vi "create.vi"(8 "error in (no error)":errorcluster) -> (0 "error out":errorcluster, 3 "system out":refnum<class "system.lvclass">)   [LabVIEW 2021, in "system.lvclass"]
uses:
  system.lvclass
  system.lvclass/system.ctl
  system.threading/system.threading.lvclass
  system.logging/system.logging.lvclass
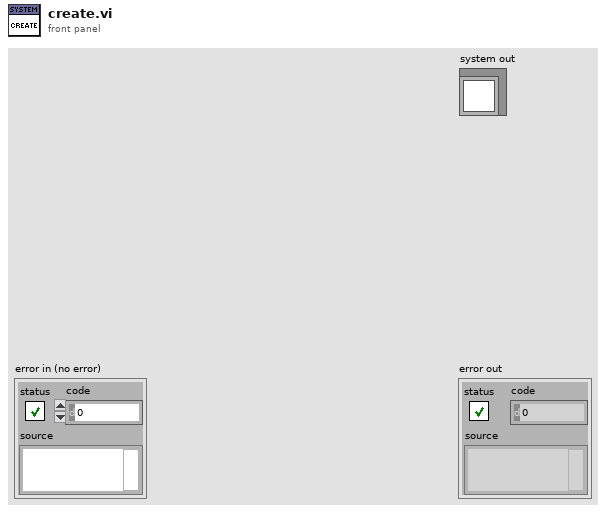
[diagram p1: front panel]
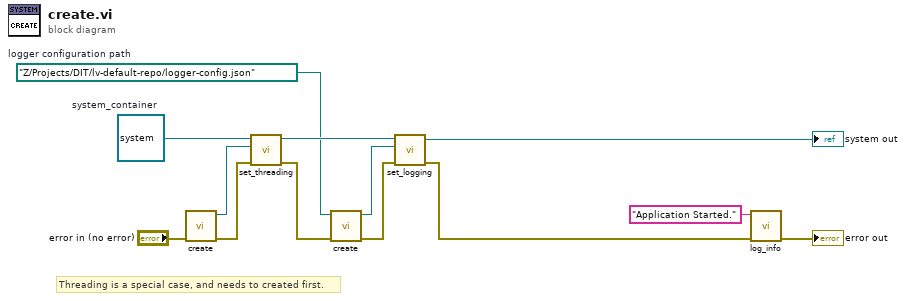
[diagram p0: block diagram]
diagram:
  w4 = path "Z:/Projects/DIT/lv-default-repo/logger-config.json"  # logger configuration path
  w10 = refnum<class "system.lvclass"> refnum  # system_container
  # "Threading is a special case, and needs to created first."
  n1 = call "create.vi"("error in (no error)"="error in (no error)") -> ("error out"=w12:errorcluster, "system.threading out"=w11:refnum<class "system.threading.lvclass">)  [unwired: 9 in]
  n2 = call "set_threading.vi"("error in (no error)"=w12, "system.threading.lvclass"=w11, "system in"=w10) -> ("error out"=w9:errorcluster, "system out"=w6:refnum<class "system.lvclass">)  [unwired: 7 in]
  n3 = call "create.vi"("error in (no error)"=w9, "path"=w4) -> ("error out"=w8:errorcluster, "logging"=w7:refnum<class "system.logging.lvclass">)  [unwired: 8 in]
  n4 = call "set_logging.vi"("error in (no error)"=w8, "system.logging.lvclass"=w7, "system in"=w6) -> ("error out"=w3:errorcluster, "system out"=→"system out":refnum<class "system.lvclass">)  [unwired: 7 in]
  n5 = call "log_info.vi"("error in (no error)"=w3, "message"="Application Started.") -> ("error out"=→"error out":errorcluster)  [unwired: 9 in]
